vi "ConfigureHallsensorSensorType.vi"(4 "error in (no error)":errorcluster, 5 "SensorType":u16(ring) items=["Hall sensors"], 6 "hallsensor configuration":cluster{"invertedPolarity":i32}, 7 "axis in":cluster{"keyHandle":u32, "nodeId":u16}={"keyHandle"=0, "nodeId"=1}) -> (0 "error out":errorcluster, 3 "axis out":cluster{"keyHandle":u32, "nodeId":u16}={"keyHandle"=0, "nodeId"=1})   [LabVIEW 2019, in "maxonEPOS.lvlib"]
doc: "<B>ConfigureHallsensorSensorType</B> writes the value for sensor type 'hallsensor' to the device. Parameters from the sensor type can be set."
uses:
  Examples/maxonEPOS.lvlib
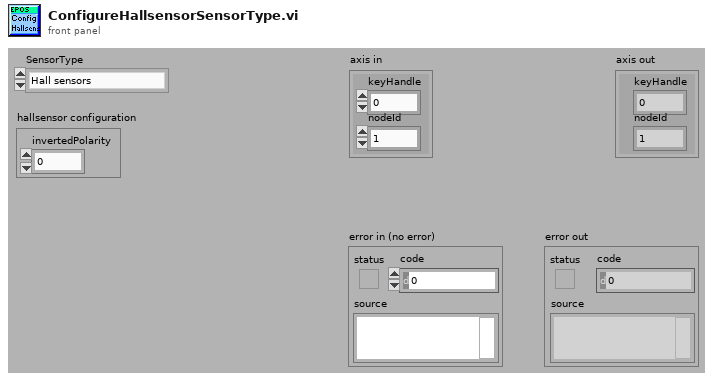
[diagram p1: front panel]
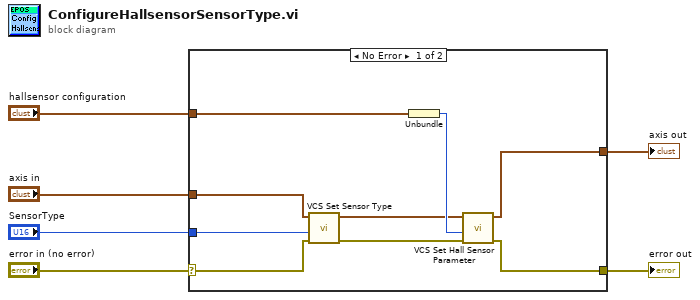
[diagram p0: block diagram]
diagram:
  n1 = case shown="No Error" "error in (no error)" {
    selector: "error in (no error)" -> [w14 w17]
    tunnel: [w9 w17] -> w5
    tunnel: [w10 w16] -> w4
    tunnel: "axis in" -> [w15 w16]
    tunnel: "hallsensor configuration" -> [w13 _]
    tunnel: "SensorType" -> [w7 _]
    frame No Error {
      n2 = call "VCS Set Sensor Type.vi"("error in (no error)"=w14, "SensorType"=w7, "axis in"=w15) -> ("error out"=w8:errorcluster, "axis out"=w11:cluster{"keyHandle":u32, "nodeId":u16})  [unwired: 7 in]
      n3 = Unbundle(w13) -> ("invertedPolarity"=w12:i32)
      n4 = call "VCS Set Hall Sensor Parameter.vi"("error in (no error)"=w8, "invertedPolarity"=w12, "axis in"=w11) -> ("error out"=w9:errorcluster, "axis out"=w10:cluster{"keyHandle":u32, "nodeId":u16})  [unwired: 7 in]
    }
    frame Error {
    }
  }
  "error out" <- w5
  "axis out" <- w4
